vi "TranslateStmCmd.vi"(10 "String":string, 11 "Buffer":string) -> (1 "”µÖµ":u16, 2 "î‘B":T1(ring))   [LabVIEW 2018]
panel:
  out "Numeric":u8 format="%x"
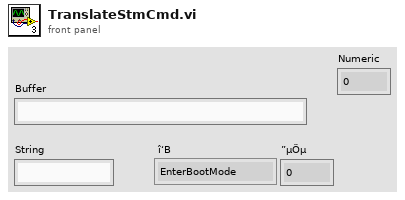
[diagram p1: front panel]
types:
  T1 = enum16{"EnterBootMode", "StartToProgram", "ProgramLineOK", "ProgramAllOk", "Error", "NULL"}
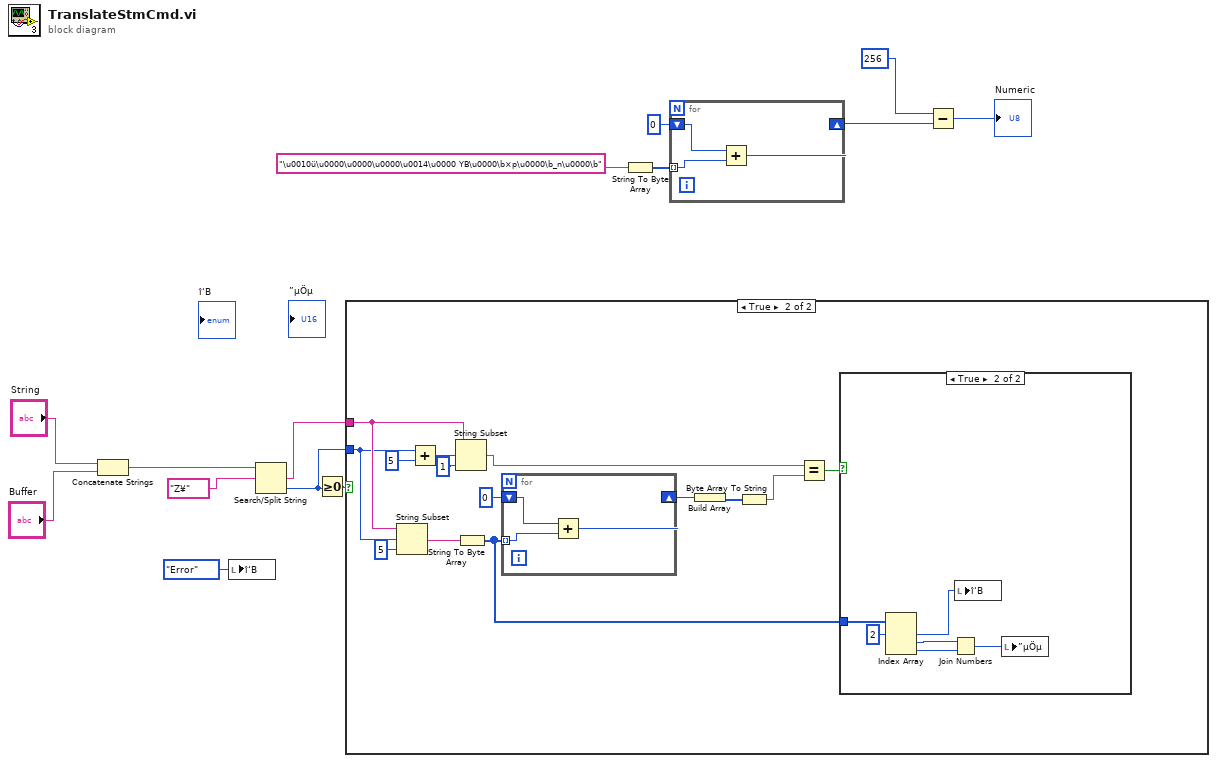
[diagram p0: block diagram]
diagram:
  n1 = Concatenate Strings("String", "Buffer") -> (w12:string)
  n2 = local write "î‘B"(T1."Error" ("î‘B")) -> ()
  n3 = Search/Split String(string=w12, search string/char (-)="Z¥" ("y")) -> (match + rest of string=w9:string, offset of match=w8:i32)  [unwired: 1 in, 1 out]
  n4 = Greater Or Equal To 0?(x=w8) -> (x >= 0?=w10:bool)
  n5 = case shown="True" w10 {
    tunnel: w9 -> [_ w25]
    tunnel: w8 -> [_ w24]
    frame False {
    }
    frame True {
      n6 = String Subset(string=w25, offset (0)=w24, length (rest)=5 ("length (rest)")) -> (substring=w20:string)
      n7 = Add(x=w24, y=5) -> (x+y=w27:i32)
      n8 = String Subset(string=w25, offset (0)=w27, length (rest)=1 ("length (rest)")) -> (substring=w18:string)
      n9 = String To Byte Array(string=w20) -> (unsigned byte array=w15:u8[])
      n10 = for {
        shift-right: [w36] -> w21
        shift-left: u8 0 -> [w37]
        tunnel: w15 -> [w35] mode=indexing
        n11 = Add(x=w37, y=w35) -> (x+y=w36:u8)
      }
      n12 = Build Array(w21) -> (w22:u8[])
      n13 = Byte Array To String(unsigned byte array=w22) -> (string=w17:string)
      n14 = Equal?(x=w18, y=w17) -> (x = y?=w16:bool)
      n15 = case shown="True" w16 {
        tunnel: w15 -> [_ w34]
        frame False {
        }
        frame True {
          n16 = Index Array(array=w34, index #1=2 ("index")) -> (element #1=w32:u8, element #2=w31:u8, element #3=w30:u8)  [unwired: 2 in]
          n17 = Join Numbers(hi=w31, lo=w30) -> ((hi.lo)=w29:u16)
          n18 = local write "î‘B"(w32) -> ()
          n19 = local write "”µÖµ"(w29) -> ()
        }
      }
    }
  }
  n20 = String To Byte Array(string="\u0010ü\u0000\u0000\u0000\u0014\u0000 YB\u0000\b×p\u0000\b_n\u0000\b") -> (unsigned byte array=w6:u8[])
  n21 = for {
    shift-right: [w39] -> w2
    shift-left: u8 0 -> [w40]
    tunnel: w6 -> [w38] mode=indexing
    n22 = Add(x=w40, y=w38) -> (x+y=w39:u8)
  }
  n23 = Subtract(x=256, y=w2) -> (x-y=→"Numeric":i32)
